vi "Close.vi"(8 "error in (no error)":errorcluster, 11 "NI Switch in":refnum<class "NI Switch.lvclass">) -> (0 "error out":errorcluster, 3 "NI Switch out":refnum<class "NI Switch.lvclass">)   [LabVIEW 2019, in "Concrete.lvlib" / "NI Switch.lvclass"]
uses:
  NI Switch.lvclass
  NI Switch.lvclass/NI Switch.ctl
  Harware Abstraction/Switch/Switch.lvclass
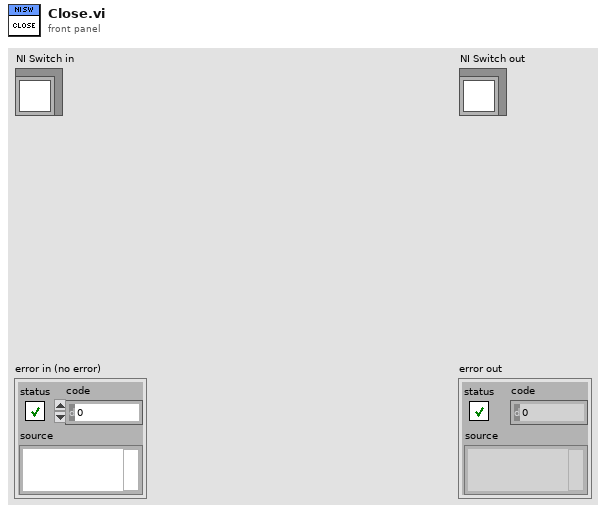
[diagram p1: front panel]
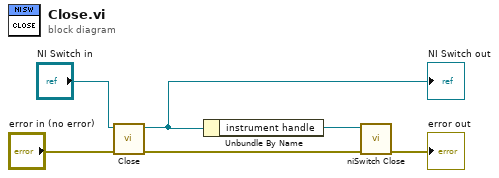
[diagram p0: block diagram]
diagram:
  n1 = call-parent "Close.vi"("error in (no error)"="error in (no error)", "Instrument in"="NI Switch in") -> ("error out"=w4:errorcluster, "Instrument out"=w2:refnum<class "NI Switch.lvclass">)  [unwired: 8 in]
  "NI Switch out" <- w2
  n2 = Unbundle By Name(w2) -> ("instrument handle"=w1:refnum<k15>)
  n3 = call <instrlib>:"niSwitch Close.vi"("error in (no error)"=w4, "instrument handle"=w1) -> ("error out"=→"error out":errorcluster)  [unwired: 9 in]
